vi "PartMaking.vi"(0 "reference in":refnum<class "Director.lvclass">, 5 "error in (no error)":errorcluster) -> (14 "reference out":refnum<class "Director.lvclass">, 19 "error out":errorcluster)   [LabVIEW 2013, in "Director.lvclass"]
uses:
  Director.lvclass
  Part_class/Part.lvclass
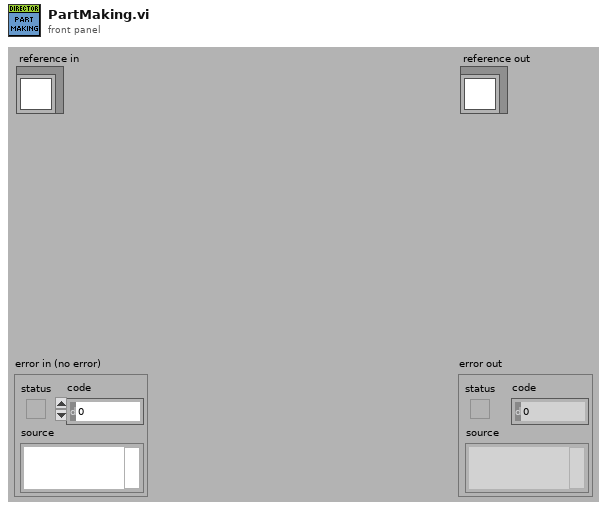
[diagram p1: front panel]
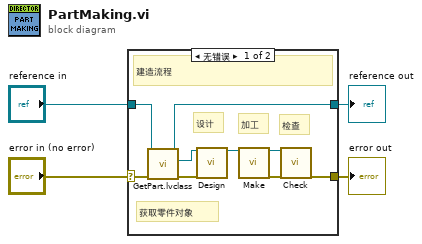
[diagram p0: block diagram]
diagram:
  n1 = case shown="无错误" "error in (no error)" {
    selector: "error in (no error)" -> [w12 w15]
    tunnel: [w6 w15] -> w3
    tunnel: [w5 w14] -> w1
    tunnel: "reference in" -> [w13 w14]
    frame No Error {
      # "检查"
      # "加工"
      # "设计"
      # "获取零件对象"
      # "建造流程"
      n2 = call "GetPart.lvclass.vi"("error in (no error)"=w12, "reference in"=w13) -> ("error out"=w10:errorcluster, "Part.lvclass"=w11:refnum<class "Part.lvclass">, "reference out"=w5:refnum<class "Director.lvclass">)  [unwired: 7 in]
      n3 = call-dynamic "Design.vi"("reference in"=w11, "error in (no error)"=w10) -> ("reference out"=w9:refnum<class "Part.lvclass">)  [unwired: 16 in, 1 out]
      n4 = call-dynamic "Make.vi"("reference in"=w9) -> ("reference out"=w8:refnum<class "Part.lvclass">, "error out"=w7:errorcluster)  [unwired: 17 in]
      n5 = call-dynamic "Check.vi"("reference in"=w8, "error in (no error)"=w7) -> ("error out"=w6:errorcluster)  [unwired: 16 in, 1 out]
    }
    frame Error {
    }
  }
  "error out" <- w3
  "reference out" <- w1
